vi "test-runge-kutta-time-varying-callback.vi"(9 "Y":T1, 10 "T":dbl, 11 "Variant":variant) -> (0 "Error":bool, 3 "output matrix":T1)   [LabVIEW 2019]
uses:
  <vilib>/Analysis/Matrix/Datatypes/RealMatrix.ctl
  <vilib>/Rock Robotics/WPI/ThirdParty/JAS_Junk/TrajLib/MatBuilder_Create.vi
  <vilib>/Rock Robotics/WPI/ThirdParty/JAS_Junk/TrajLib/Trajectory_Library.lvlib
  <vilib>/Analysis/Matrix/NI_Matrix.lvlib
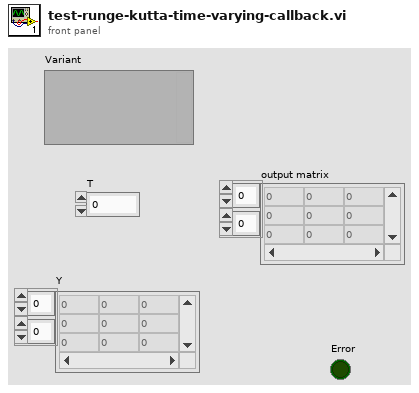
[diagram p1: front panel]
types:
  T1 = typedef "NI_Matrix.lvlib/RealMatrix.ctl" = dbl[][]
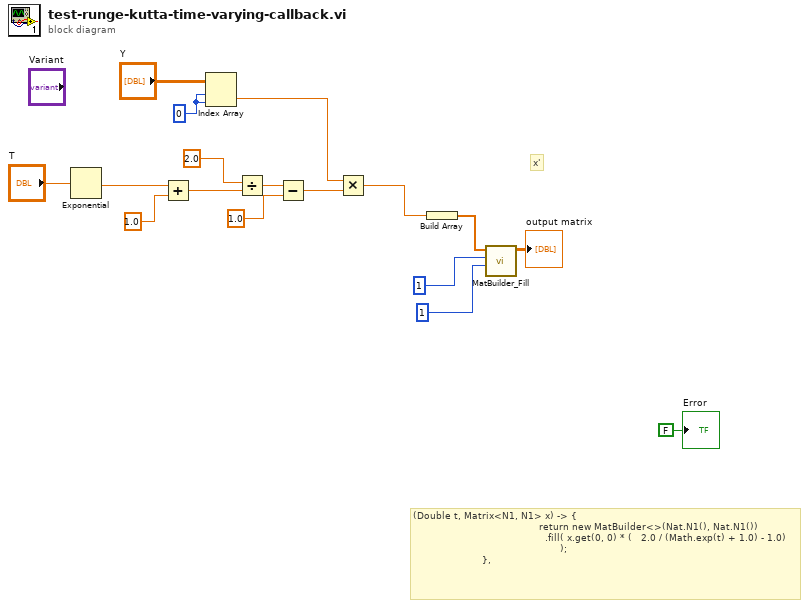
[diagram p0: block diagram]
diagram:
  w7 = 0 ("index (row)")
  # "x'"
  # "(Double t, Matrix<N1, N1> x) -> {\n                                          return new MatBuilder<>(Nat.N1(), Nat.N1())\n                                            .fill( x.get(0, 0) * (   2.0 / (Math.exp(t) + 1.0) - 1.0)\n                                                 );\n                       },"
  n1 = Exponential(1:"T") -> (0:w14:dbl)
  n2 = Add(x=w14, y=1.0) -> (x+y=w8:dbl)
  n3 = Index Array(array="Y", index (row)=w7, index (col)=w7) -> (element=w2:dbl)
  n4 = Divide(x=2.0, y=w8) -> (x/y=w5:dbl)
  n5 = Subtract(x=w5, y=1.0) -> (x-y=w3:dbl)
  n6 = Multiply(x=w2, y=w3) -> (x*y=w1:dbl)
  n7 = Build Array(w1) -> (w12:dbl[])
  n8 = call <vilib>:"MatBuilder_Fill.vi"("Columns"=1, "Rows"=1, "Value List"=w12) -> ("output matrix"=→"output matrix":T1)  [unwired: 8 in]
  "Error" <- FALSE ("Error")
